vi "Autonomous Independent.vi"() -> ()   [LabVIEW 2014]
doc: "This VI is called when autonomous begins, and will automatically be terminated when autonomous ends. You can carry out timed or sensor driven robot movement independently without needing to return to the caller."
uses:
  Robot Global Data.vi
  <vilib>/Rock Robotics/WPI/RobotDrive/WPI_RobotDriveMecanumDrive_Cartesian.vi
  <vilib>/addons/control/pid/NI_PID_pid.lvlib
  <vilib>/addons/control/pid/pid.llb/PID (DBL).vi
  <vilib>/Rock Robotics/WPI/Relay/WPI_RelayValue.ctl
panel:
  out "Motor Outputs 2":dbl(graph)=0.07468179223935595
  in  "Target Center Gains":T1={"proportional gain (Kc)"=0.2, "integral time (Ti, min)"=0.0, "derivative time (Td, min)"=0.4} {"derivative time (Td, min)" format="%#.6g"; "integral time (Ti, min)" format="%#.6g"; "proportional gain (Kc)" format="%#.6g"}
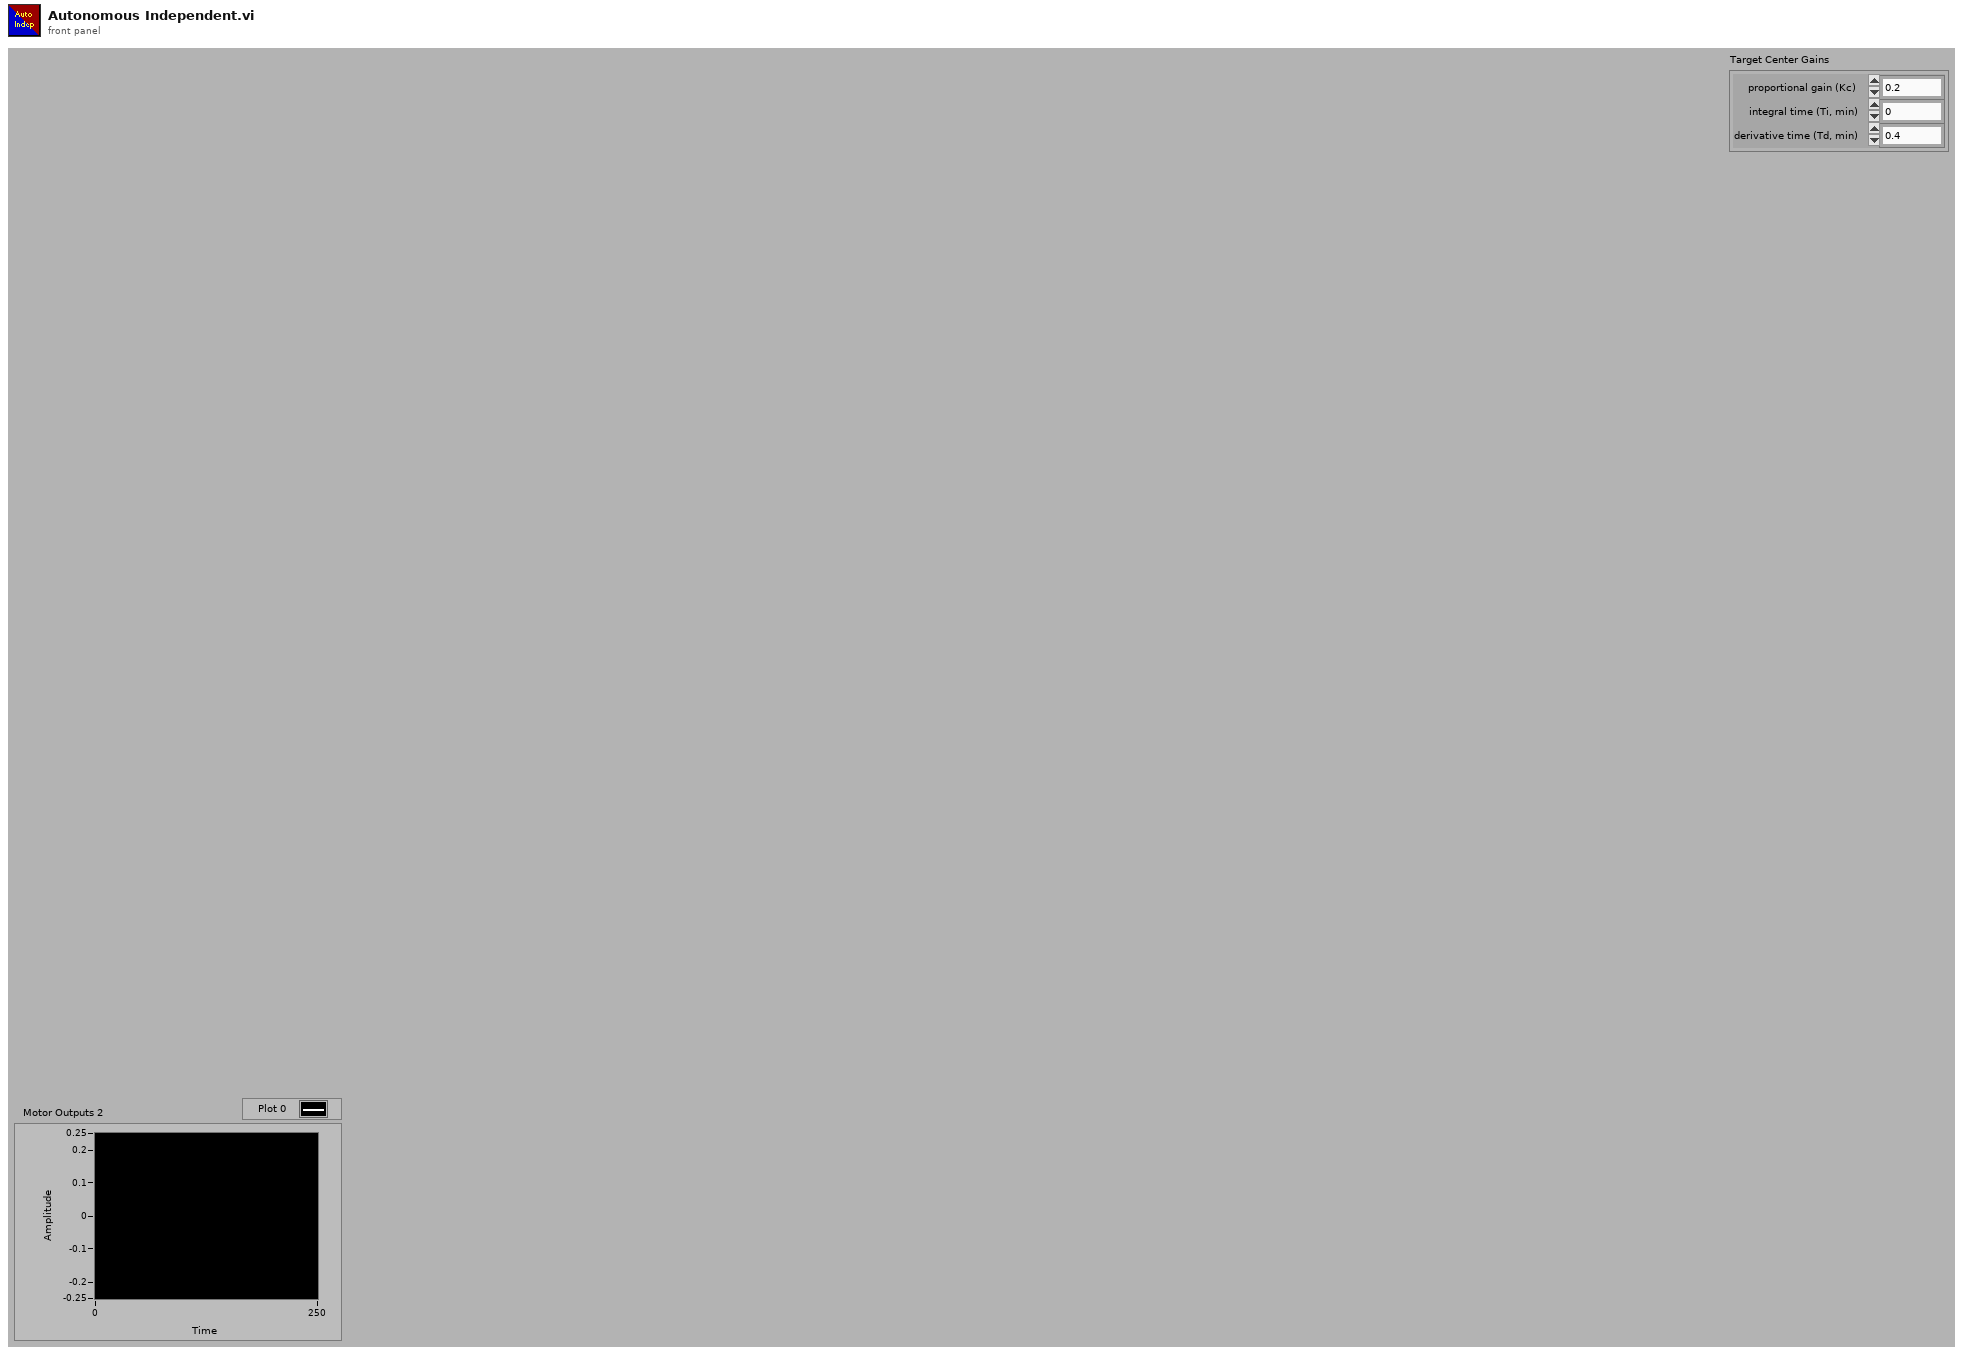
[diagram p1: front panel]
types:
  T1 = cluster{"proportional gain (Kc)":dbl, "integral time (Ti, min)":dbl, "derivative time (Td, min)":dbl}
  T2 = typedef "WPI_RelayValue.ctl" = enum16{"Off", "On", "Forward", "Reverse"}
  T3 = typedef "WPI_RelayDevRef.ctl" = cluster{"DevStatus":errorcluster, "Relay Channel":T4, "Digital Module":T5, "Relay Direction":T6}
  T4 = typedef "FPGA_DIORelayChannel.ctl" = enum8{"Relay 1", "Relay 2", "Relay 3", "Relay 4", "Relay 5", "Relay 6", "Relay 7", "Relay 8", "Invalid"}
  T5 = typedef "FPGA_TypedefDigitalModule.ctl" = enum16{"Digital Module 1", "Digital Module 2"}
  T6 = typedef "WPI_RelayDirection.ctl" = enum16{"Both directions", "Forward only", "Reverse only"}
  T7 = typedef "WPI_RobotDriveDevRef.ctl" = cluster{"DevStatus":errorcluster, "Motors[]":T8[], "Square Inputs":bool, "Max Output":dbl, "Isochronous":bool}
  T8 = typedef "WPI_MotorControlDeviceRef.ctl" = cluster{"DeviceStatus":errorcluster, "Type":enum16{"PWM", "CAN"}, "PWM":cluster{"Digital Module":T5, "PWM Channel":T9, "DeadBand":T10}, "CAN":cluster{"Device Number":u8, "Control Mode":T11, "Semaphore":T12, "Max Vout":dbl}, "Invert":bool, "TransformRef":T13, "InvTransformRef":T13}
  T9 = typedef "FPGA_DIOPWMChannel.ctl" = enum8{"PWM 1", "PWM 2", "PWM 3", "PWM 4", "PWM 5", "PWM 6", "PWM 7", "PWM 8", "PWM 9", "PWM 10", "Invalid"}
  T10 = typedef "WPI_PWMDeadband.ctl" = cluster{"Name":string, "maxPositivePwm":i32, "minPositivePwm":i32, "centerPwm":i32, "maxNegativePwm":i32, "minNegativePwm":i32, "angularRange":u16}
  T11 = typedef "WPI_CANJaguar_ControlMode.ctl" = enum8{"Percent VBus", "Current", "Speed", "Position", "Voltage"}
  T12 = typedef "Semaphore RefNum" = refnum<k1>
  T13 = typedef "WPI_PWMTransform_ConPane.ctl" = refnum<vi>
  T14 = typedef "WPI_JoystickDevRef.ctl" = cluster{"Device":T15}
  T15 = typedef "WPI_JoystickDeviceEnum.ctl" = enum16{"USB 1", "USB 2", "USB 3", "USB 4", "Kinect 1", "Kinect 2"}
  T16 = cluster{"axis 1 (x)":dbl, "axis 2 (y)":dbl, "axis 3 (throttle)":dbl, "axis 4":dbl, "axis 5":dbl, "axis 6":dbl}
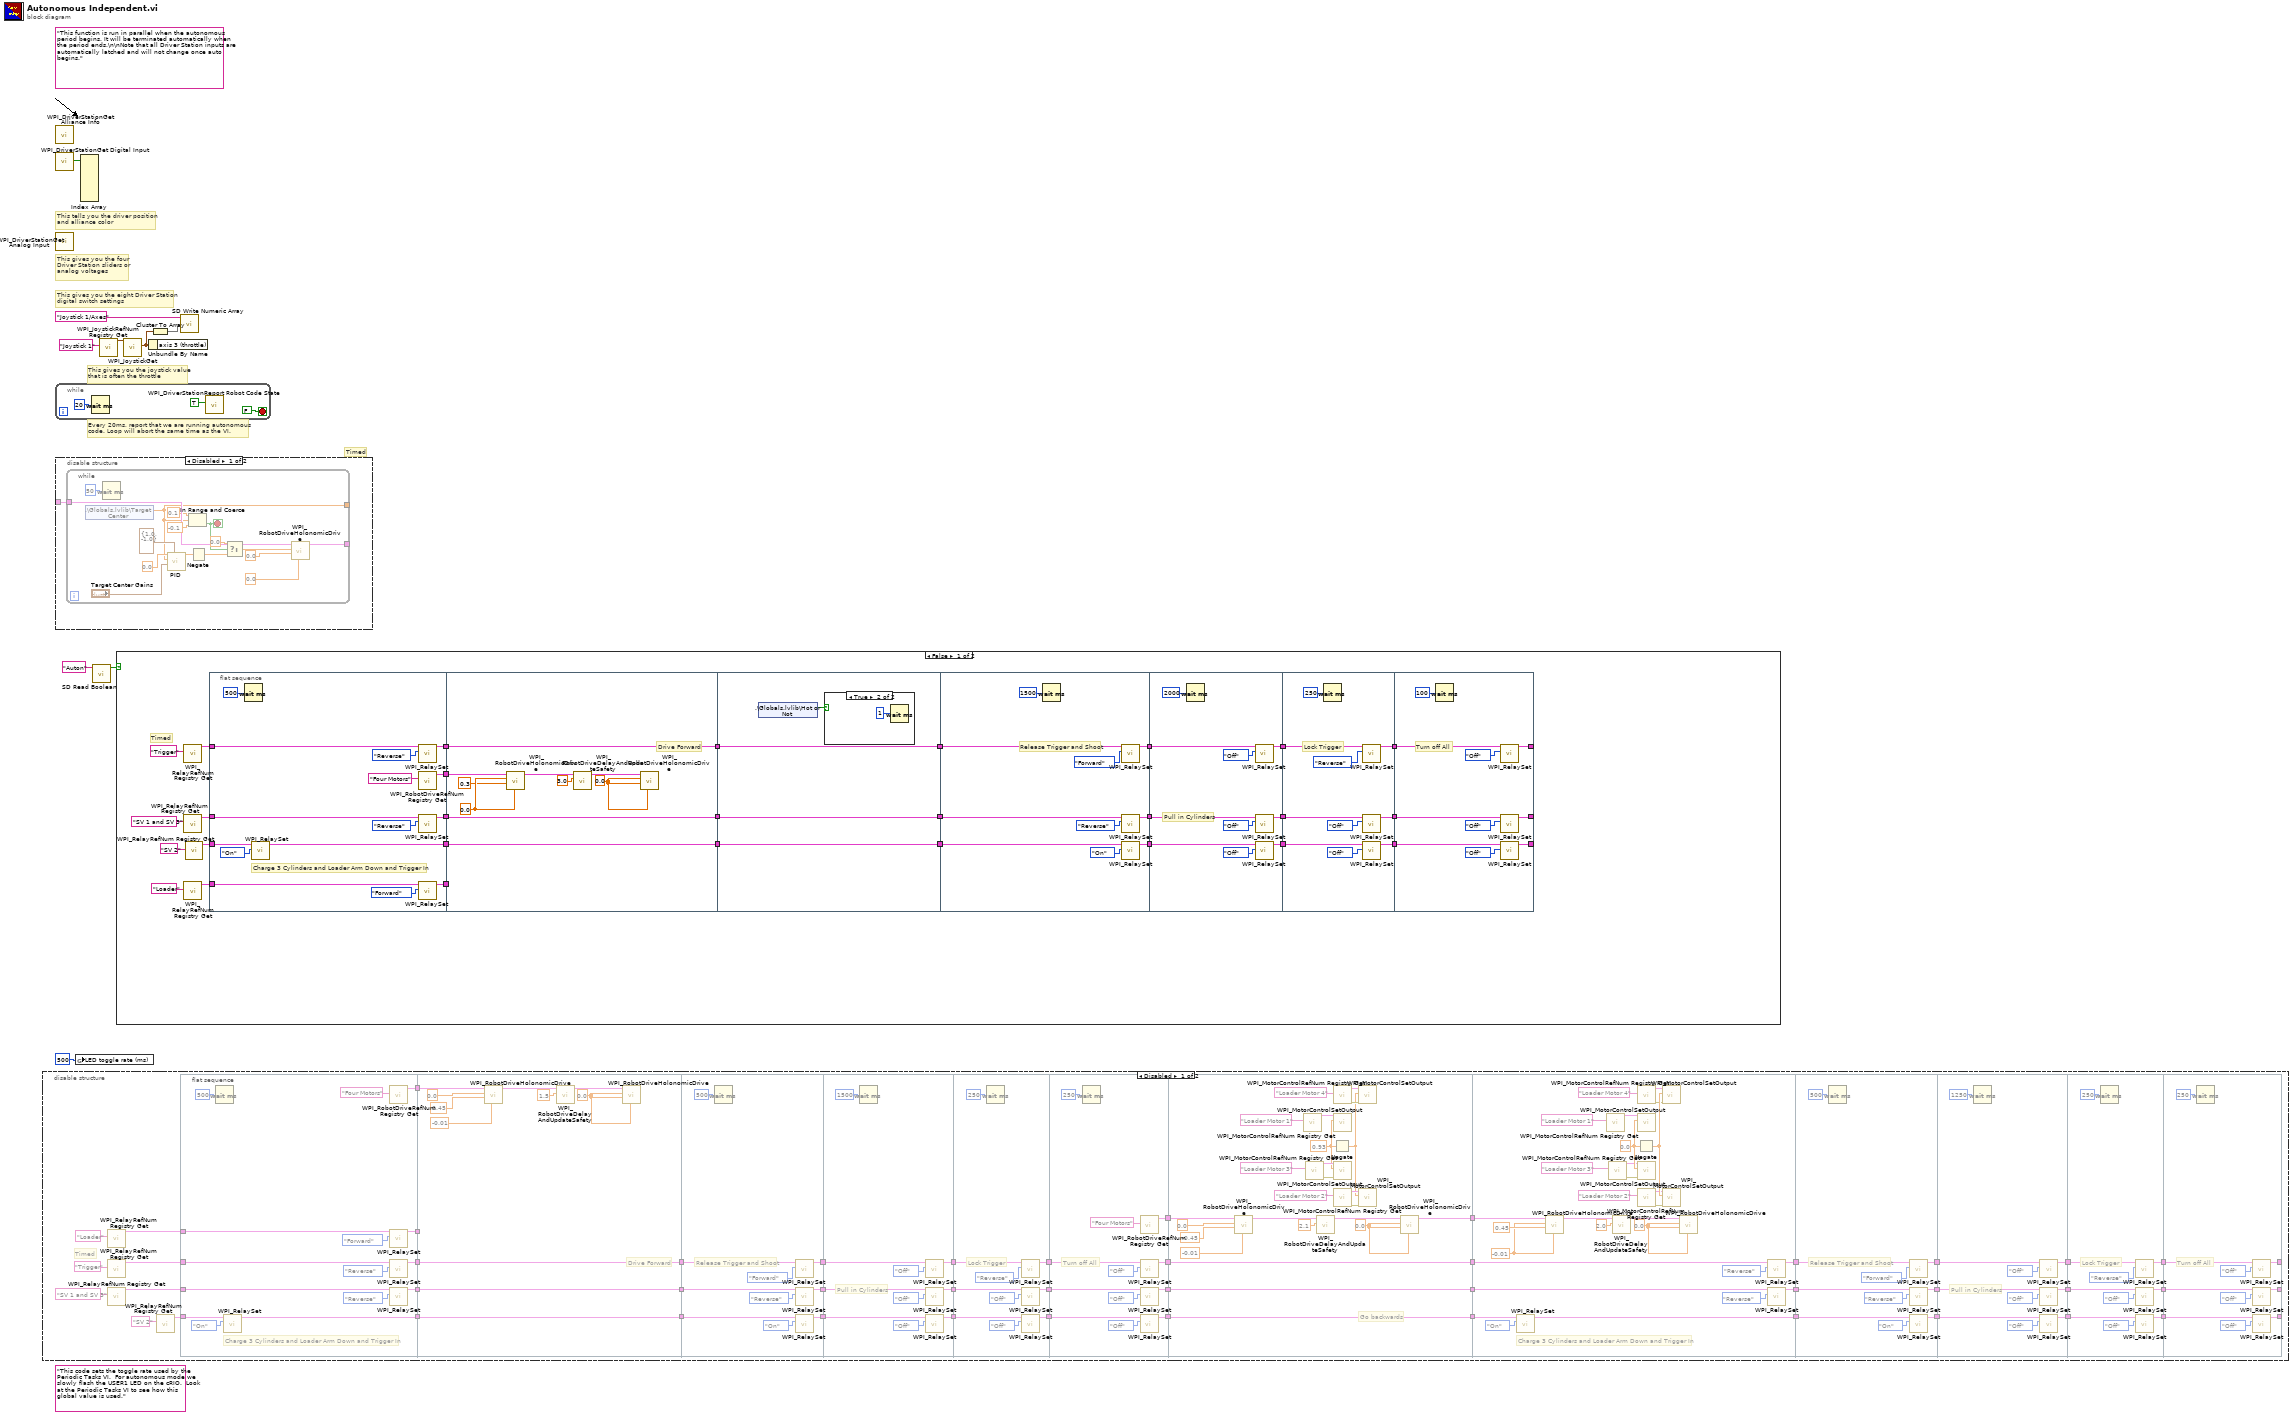
[diagram p0: block diagram]
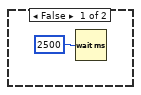
[diagram p2: hidden frame]
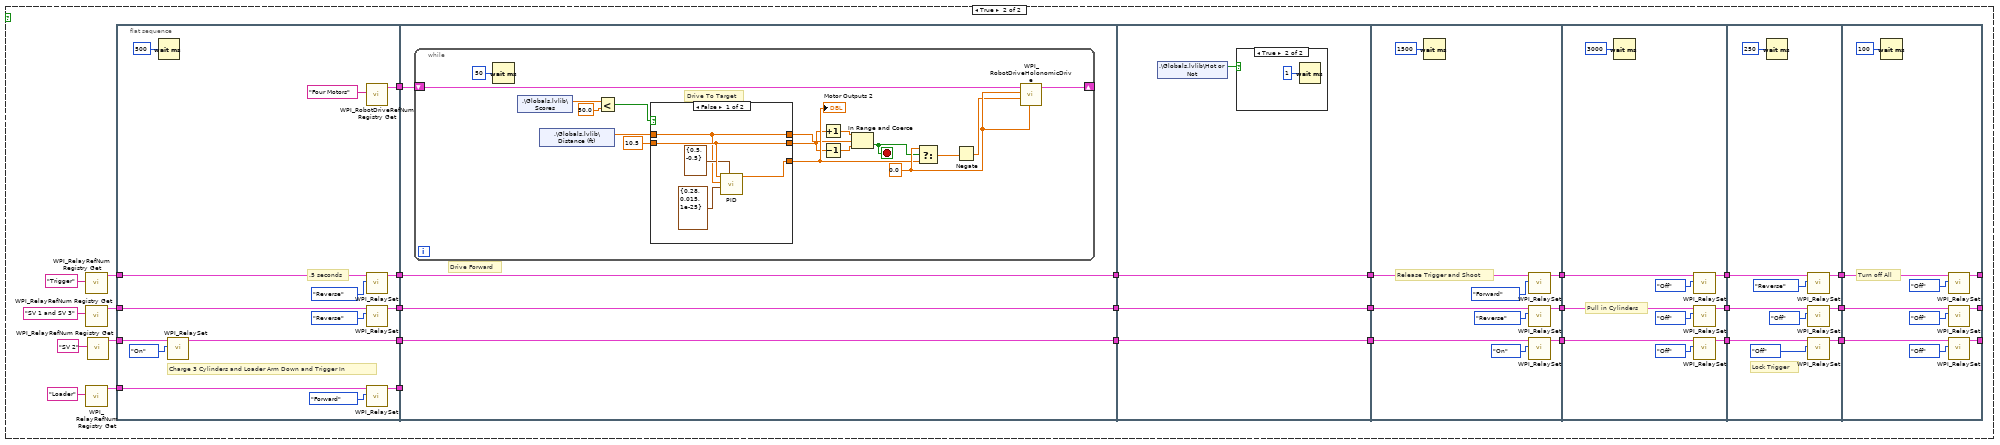
[diagram p3: hidden frame]
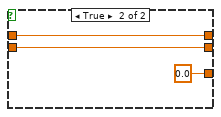
[diagram p4: hidden frame]
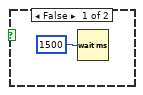
[diagram p5: hidden frame]
diagram:
  (unwired) "This code sets the toggle rate used by the Periodic Tasks VI.  For autonomous mode we slowly flash the USER1 LED on the cRIO.  Look at the Periodic Tasks VI to see how this global value is used."
  (unwired) "This function is run in parallel when the autonomous period begins. It will be terminated automatically when the period ends.\n\nNote that all Driver Station inputs are automatically latched and will not change once auto begins."
  # "Timed"
  # "Every 20ms, report that we are running autonomous\ncode. Loop will abort the same time as the VI."
  # "This gives you the joystick value\nthat is often the throttle"
  # "This tells you the driver position\nand alliance color"
  # "This gives you the eight Driver Station\ndigital switch settings"
  # "This gives you the four\nDriver Station sliders or\nanalog voltages"
  n1 = disable-structure shown="Disabled" {
    frame Disabled {
      # "Timed"
      n2 = call <vilib>:"WPI_RelayRefNum Registry Get.vi"("refnum name"="Loader") -> ("RelayDevRef"=w14:T3)  [unwired: 9 in, 1 out]
      n3 = call <vilib>:"WPI_RelayRefNum Registry Get.vi"("refnum name"="Trigger") -> ("RelayDevRef"=w16:T3)  [unwired: 9 in, 1 out]
      n4 = call <vilib>:"WPI_RelayRefNum Registry Get.vi"("refnum name"="SV 1 and SV 3") -> ("RelayDevRef"=w12:T3)  [unwired: 9 in, 1 out]
      n5 = call <vilib>:"WPI_RelayRefNum Registry Get.vi"("refnum name"="SV 2") -> ("RelayDevRef"=w10:T3)  [unwired: 9 in, 1 out]
      n6 = flat-sequence {
        tunnel: [w64] -> w54
        tunnel: [w63] -> w53
        tunnel: [w62] -> w52
        tunnel: [w61] -> w51
        tunnel: [w59] -> w50
        tunnel: w16 -> [w58]
        tunnel: w14 -> [w57]
        tunnel: w12 -> [w56]
        tunnel: w10 -> [w55]
        tunnel: w54 -> [_]
        tunnel: w53 -> [w80]
        tunnel: w52 -> [w79]
        tunnel: w51 -> [w78]
        tunnel: w50 -> [w73]
        tunnel: [w80] -> w47
        tunnel: [w79] -> w48
        tunnel: [w78] -> w49
        tunnel: [w83] -> w46
        tunnel: [w82] -> w45
        tunnel: [w81] -> w44
        tunnel: w49 -> [w84]
        tunnel: w48 -> [w85]
        tunnel: w47 -> [w86]
        tunnel: w46 -> [w96]
        tunnel: w45 -> [w95]
        tunnel: w44 -> [w94]
        tunnel: [w93] -> w43
        tunnel: [w92] -> w42
        tunnel: [w91] -> w41
        tunnel: w43 -> [w106]
        tunnel: w42 -> [w105]
        tunnel: w41 -> [w104]
        tunnel: [w103] -> w40
        tunnel: [w102] -> w39
        tunnel: [w101] -> w38
        tunnel: w40 -> [w118]
        tunnel: w39 -> [w117]
        tunnel: w38 -> [w116]
        tunnel: [w115] -> w37
        tunnel: [w114] -> w36
        tunnel: [w113] -> w35
        tunnel: [w111] -> w34
        tunnel: w37 -> [w147]
        tunnel: w36 -> [w146]
        tunnel: w35 -> [w145]
        tunnel: w34 -> [w138]
        tunnel: [w147] -> w30
        tunnel: [w146] -> w31
        tunnel: [w145] -> w32
        tunnel: [w124] -> w33
        tunnel: [w176] -> w29
        tunnel: [w175] -> w28
        tunnel: [w174] -> w27
        tunnel: w33 -> [w150]
        tunnel: w32 -> [w155]
        tunnel: w31 -> [w156]
        tunnel: w30 -> [w157]
        tunnel: w29 -> [w180]
        tunnel: w28 -> [w182]
        tunnel: w27 -> [w178]
        tunnel: [w181] -> w26
        tunnel: [w179] -> w25
        tunnel: [w177] -> w24
        tunnel: w26 -> [w192]
        tunnel: w25 -> [w191]
        tunnel: w24 -> [w190]
        tunnel: [w189] -> w23
        tunnel: [w188] -> w22
        tunnel: [w187] -> w21
        tunnel: w23 -> [w202]
        tunnel: w22 -> [w201]
        tunnel: w21 -> [w200]
        tunnel: [w199] -> w20
        tunnel: [w198] -> w19
        tunnel: [w197] -> w18
        tunnel: w20 -> [w212]
        tunnel: w19 -> [w211]
        tunnel: w18 -> [w210]
        tunnel: [w209] -> _
        tunnel: [w208] -> _
        tunnel: [w207] -> _
        frame #0 {
          # "Charge 3 Cylinders and Loader Arm Down and Trigger In"
          n7 = Wait (ms)(milliseconds to wait=u32 500) -> ()  [unwired: 1 out]
          n8 = call <vilib>:"WPI_RelaySet.vi"("RelayValue"=WPI_RelayValue."On", "RelayDevRef"=w55) -> ("RelayDevRef"=w63:T3)  [unwired: 8 in, 1 out]
          n9 = call <vilib>:"WPI_RobotDriveRefNum Registry Get.vi"("refnum name"="Four Motors") -> ("RobotDriveDevRef"=w59:T7)  [unwired: 1 in, 9 out]
          n10 = call <vilib>:"WPI_RelaySet.vi"("RelayValue"=WPI_RelayValue."Forward", "RelayDevRef"=w57) -> ("RelayDevRef"=w64:T3)  [unwired: 8 in, 1 out]
          n11 = call <vilib>:"WPI_RelaySet.vi"("RelayValue"=WPI_RelayValue."Reverse", "RelayDevRef"=w58) -> ("RelayDevRef"=w62:T3)  [unwired: 8 in, 1 out]
          n12 = call <vilib>:"WPI_RelaySet.vi"("RelayValue"=WPI_RelayValue."Reverse", "RelayDevRef"=w56) -> ("RelayDevRef"=w61:T3)  [unwired: 8 in, 1 out]
        }
        frame #1 {
          w74 = 0.0 ("Y")
          # "Drive Forward"
          n13 = call-poly <vilib>:"WPI_RobotDriveHolonomicDrive.vi"("Rotation"=-0.01, "Y"=0.45, "X"=0.0 ("Y"), "RobotDriveDevRef"=w73) -> ("RobotDriveDevRef"=w77:T7)  [unwired: 5 in, 2 out]
          n14 = call <vilib>:"WPI_RobotDriveDelayAndUpdateSafety.vi"("Delay (s)"=1.5, "RobotDriveDevRef"=w77) -> ("RobotDriveDevRef 2"=w75:T7)  [unwired: 8 in, 1 out]
          n15 = call-poly <vilib>:"WPI_RobotDriveHolonomicDrive.vi"("Rotation"=w74, "Y"=w74, "X"=w74, "RobotDriveDevRef"=w75) -> ()  [unwired: 5 in, 3 out]
        }
        frame #2 {
          # "Release Trigger and Shoot"
          n16 = Wait (ms)(milliseconds to wait=u32 500) -> ()  [unwired: 1 out]
          n17 = call <vilib>:"WPI_RelaySet.vi"("RelayValue"=WPI_RelayValue."Forward", "RelayDevRef"=w85) -> ("RelayDevRef"=w82:T3)  [unwired: 8 in, 1 out]
          n18 = call <vilib>:"WPI_RelaySet.vi"("RelayValue"=WPI_RelayValue."Reverse", "RelayDevRef"=w84) -> ("RelayDevRef"=w81:T3)  [unwired: 8 in, 1 out]
          n19 = call <vilib>:"WPI_RelaySet.vi"("RelayValue"=WPI_RelayValue."On", "RelayDevRef"=w86) -> ("RelayDevRef"=w83:T3)  [unwired: 8 in, 1 out]
        }
        frame #3 {
          # "Pull in Cylinders"
          n20 = Wait (ms)(milliseconds to wait=u32 1500) -> ()  [unwired: 1 out]
          n21 = call <vilib>:"WPI_RelaySet.vi"("RelayValue"=WPI_RelayValue."Off", "RelayDevRef"=w95) -> ("RelayDevRef"=w92:T3)  [unwired: 8 in, 1 out]
          n22 = call <vilib>:"WPI_RelaySet.vi"("RelayValue"=WPI_RelayValue."Off", "RelayDevRef"=w94) -> ("RelayDevRef"=w91:T3)  [unwired: 8 in, 1 out]
          n23 = call <vilib>:"WPI_RelaySet.vi"("RelayValue"=WPI_RelayValue."Off", "RelayDevRef"=w96) -> ("RelayDevRef"=w93:T3)  [unwired: 8 in, 1 out]
        }
        frame #4 {
          # "Lock Trigger"
          n24 = Wait (ms)(milliseconds to wait=u32 250) -> ()  [unwired: 1 out]
          n25 = call <vilib>:"WPI_RelaySet.vi"("RelayValue"=WPI_RelayValue."Reverse", "RelayDevRef"=w105) -> ("RelayDevRef"=w102:T3)  [unwired: 8 in, 1 out]
          n26 = call <vilib>:"WPI_RelaySet.vi"("RelayValue"=WPI_RelayValue."Off", "RelayDevRef"=w104) -> ("RelayDevRef"=w101:T3)  [unwired: 8 in, 1 out]
          n27 = call <vilib>:"WPI_RelaySet.vi"("RelayValue"=WPI_RelayValue."Off", "RelayDevRef"=w106) -> ("RelayDevRef"=w103:T3)  [unwired: 8 in, 1 out]
        }
        frame #5 {
          # "Turn off All"
          n28 = Wait (ms)(milliseconds to wait=u32 250) -> ()  [unwired: 1 out]
          n29 = call <vilib>:"WPI_RobotDriveRefNum Registry Get.vi"("refnum name"="Four Motors") -> ("RobotDriveDevRef"=w111:T7)  [unwired: 1 in, 9 out]
          n30 = call <vilib>:"WPI_RelaySet.vi"("RelayValue"=WPI_RelayValue."Off", "RelayDevRef"=w117) -> ("RelayDevRef"=w114:T3)  [unwired: 8 in, 1 out]
          n31 = call <vilib>:"WPI_RelaySet.vi"("RelayValue"=WPI_RelayValue."Off", "RelayDevRef"=w116) -> ("RelayDevRef"=w115:T3)  [unwired: 8 in, 1 out]
          n32 = call <vilib>:"WPI_RelaySet.vi"("RelayValue"=WPI_RelayValue."Off", "RelayDevRef"=w118) -> ("RelayDevRef"=w113:T3)  [unwired: 8 in, 1 out]
        }
        frame #6 {
          w125 = 0.93 ("t")
          w141 = 0.0 ("Y")
          # "Go backwards"
          n33 = call-poly <vilib>:"WPI_RobotDriveHolonomicDrive.vi"("Rotation"=-0.01, "Y"=-0.45, "X"=0.0 ("Y"), "RobotDriveDevRef"=w138) -> ("RobotDriveDevRef"=w144:T7)  [unwired: 5 in, 2 out]
          n34 = call <vilib>:"WPI_MotorControlRefNum Registry Get.vi"("refnum name"="Loader Motor 1") -> ("MotorControlDevRef"=w134:T8)  [unwired: 9 in, 1 out]
          n35 = call <vilib>:"WPI_MotorControlRefNum Registry Get.vi"("refnum name"="Loader Motor 3") -> ("error out"=w130:errorcluster, "MotorControlDevRef"=w131:T8)  [unwired: 9 in]
          n36 = call <vilib>:"WPI_RobotDriveDelayAndUpdateSafety.vi"("Delay (s)"=2.1, "RobotDriveDevRef"=w144) -> ("RobotDriveDevRef 2"=w142:T7)  [unwired: 8 in, 1 out]
          n37 = call <vilib>:"WPI_MotorControlRefNum Registry Get.vi"("refnum name"="Loader Motor 4") -> ("error out"=w127:errorcluster, "MotorControlDevRef"=w128:T8)  [unwired: 9 in]
          n38 = call <vilib>:"WPI_MotorControlSetOutput.vi"("Output"=w125, "MotorControlDevRef"=w134) -> ()  [unwired: 7 in, 3 out]
          n39 = Negate(x=w125) -> (-x=w126:dbl)
          n40 = call <vilib>:"WPI_MotorControlSetOutput.vi"("error in (no error)"=w130, "Output"=w125, "MotorControlDevRef"=w131) -> ()  [unwired: 6 in, 3 out]
          n41 = call <vilib>:"WPI_MotorControlRefNum Registry Get.vi"("refnum name"="Loader Motor 2") -> ("error out"=w133:errorcluster, "MotorControlDevRef"=w135:T8)  [unwired: 9 in]
          n42 = call <vilib>:"WPI_MotorControlSetOutput.vi"("error in (no error)"=w127, "Output"=w126, "MotorControlDevRef"=w128) -> ()  [unwired: 6 in, 3 out]
          n43 = call <vilib>:"WPI_MotorControlSetOutput.vi"("error in (no error)"=w133, "Output"=w126, "MotorControlDevRef"=w135) -> ()  [unwired: 6 in, 3 out]
          n44 = call-poly <vilib>:"WPI_RobotDriveHolonomicDrive.vi"("Rotation"=w141, "Y"=w141, "X"=w141, "RobotDriveDevRef"=w142) -> ("RobotDriveDevRef"=w124:T7)  [unwired: 5 in, 2 out]
        }
        frame #7 {
          w148 = -0.01 ("Y")
          w149 = 0.0 ("Y")
          w173 = 0.0 ("t")
          # "Charge 3 Cylinders and Loader Arm Down and Trigger In"
          n45 = call <vilib>:"WPI_RelaySet.vi"("RelayValue"=WPI_RelayValue."On", "RelayDevRef"=w155) -> ("RelayDevRef"=w174:T3)  [unwired: 8 in, 1 out]
          n46 = call-poly <vilib>:"WPI_RobotDriveHolonomicDrive.vi"("Rotation"=w148, "Y"=0.45, "X"=w148, "RobotDriveDevRef"=w150) -> ("RobotDriveDevRef"=w151:T7)  [unwired: 5 in, 2 out]
          n47 = call <vilib>:"WPI_MotorControlRefNum Registry Get.vi"("refnum name"="Loader Motor 1") -> ("MotorControlDevRef"=w165:T8)  [unwired: 9 in, 1 out]
          n48 = call <vilib>:"WPI_MotorControlRefNum Registry Get.vi"("refnum name"="Loader Motor 3") -> ("error out"=w169:errorcluster, "MotorControlDevRef"=w168:T8)  [unwired: 9 in]
          n49 = call <vilib>:"WPI_RobotDriveDelayAndUpdateSafety.vi"("Delay (s)"=2.0, "RobotDriveDevRef"=w151) -> ("RobotDriveDevRef 2"=w153:T7)  [unwired: 8 in, 1 out]
          n50 = call <vilib>:"WPI_MotorControlRefNum Registry Get.vi"("refnum name"="Loader Motor 4") -> ("error out"=w171:errorcluster, "MotorControlDevRef"=w161:T8)  [unwired: 9 in]
          n51 = call <vilib>:"WPI_MotorControlSetOutput.vi"("Output"=w173, "MotorControlDevRef"=w165) -> ()  [unwired: 7 in, 3 out]
          n52 = Negate(x=w173) -> (-x=w172:dbl)
          n53 = call <vilib>:"WPI_MotorControlSetOutput.vi"("error in (no error)"=w169, "Output"=w173, "MotorControlDevRef"=w168) -> ()  [unwired: 6 in, 3 out]
          n54 = call <vilib>:"WPI_MotorControlRefNum Registry Get.vi"("refnum name"="Loader Motor 2") -> ("error out"=w166:errorcluster, "MotorControlDevRef"=w164:T8)  [unwired: 9 in]
          n55 = call <vilib>:"WPI_MotorControlSetOutput.vi"("error in (no error)"=w171, "Output"=w172, "MotorControlDevRef"=w161) -> ()  [unwired: 6 in, 3 out]
          n56 = call <vilib>:"WPI_MotorControlSetOutput.vi"("error in (no error)"=w166, "Output"=w172, "MotorControlDevRef"=w164) -> ()  [unwired: 6 in, 3 out]
          n57 = call-poly <vilib>:"WPI_RobotDriveHolonomicDrive.vi"("Rotation"=w149, "Y"=w149, "X"=w149, "RobotDriveDevRef"=w153) -> ()  [unwired: 5 in, 3 out]
          n58 = call <vilib>:"WPI_RelaySet.vi"("RelayValue"=WPI_RelayValue."Reverse", "RelayDevRef"=w156) -> ("RelayDevRef"=w175:T3)  [unwired: 8 in, 1 out]
          n59 = call <vilib>:"WPI_RelaySet.vi"("RelayValue"=WPI_RelayValue."Reverse", "RelayDevRef"=w157) -> ("RelayDevRef"=w176:T3)  [unwired: 8 in, 1 out]
        }
        frame #8 {
          # "Release Trigger and Shoot"
          n60 = Wait (ms)(milliseconds to wait=u32 500) -> ()  [unwired: 1 out]
          n61 = call <vilib>:"WPI_RelaySet.vi"("RelayValue"=WPI_RelayValue."Forward", "RelayDevRef"=w182) -> ("RelayDevRef"=w181:T3)  [unwired: 8 in, 1 out]
          n62 = call <vilib>:"WPI_RelaySet.vi"("RelayValue"=WPI_RelayValue."Reverse", "RelayDevRef"=w180) -> ("RelayDevRef"=w179:T3)  [unwired: 8 in, 1 out]
          n63 = call <vilib>:"WPI_RelaySet.vi"("RelayValue"=WPI_RelayValue."On", "RelayDevRef"=w178) -> ("RelayDevRef"=w177:T3)  [unwired: 8 in, 1 out]
        }
        frame #9 {
          # "Pull in Cylinders"
          n64 = Wait (ms)(milliseconds to wait=u32 1250) -> ()  [unwired: 1 out]
          n65 = call <vilib>:"WPI_RelaySet.vi"("RelayValue"=WPI_RelayValue."Off", "RelayDevRef"=w192) -> ("RelayDevRef"=w189:T3)  [unwired: 8 in, 1 out]
          n66 = call <vilib>:"WPI_RelaySet.vi"("RelayValue"=WPI_RelayValue."Off", "RelayDevRef"=w191) -> ("RelayDevRef"=w188:T3)  [unwired: 8 in, 1 out]
          n67 = call <vilib>:"WPI_RelaySet.vi"("RelayValue"=WPI_RelayValue."Off", "RelayDevRef"=w190) -> ("RelayDevRef"=w187:T3)  [unwired: 8 in, 1 out]
        }
        frame #10 {
          # "Lock Trigger"
          n68 = Wait (ms)(milliseconds to wait=u32 250) -> ()  [unwired: 1 out]
          n69 = call <vilib>:"WPI_RelaySet.vi"("RelayValue"=WPI_RelayValue."Reverse", "RelayDevRef"=w202) -> ("RelayDevRef"=w199:T3)  [unwired: 8 in, 1 out]
          n70 = call <vilib>:"WPI_RelaySet.vi"("RelayValue"=WPI_RelayValue."Off", "RelayDevRef"=w201) -> ("RelayDevRef"=w198:T3)  [unwired: 8 in, 1 out]
          n71 = call <vilib>:"WPI_RelaySet.vi"("RelayValue"=WPI_RelayValue."Off", "RelayDevRef"=w200) -> ("RelayDevRef"=w197:T3)  [unwired: 8 in, 1 out]
        }
        frame #11 {
          # "Turn off All"
          n72 = Wait (ms)(milliseconds to wait=u32 250) -> ()  [unwired: 1 out]
          n73 = call <vilib>:"WPI_RelaySet.vi"("RelayValue"=WPI_RelayValue."Off", "RelayDevRef"=w212) -> ("RelayDevRef"=w208:T3)  [unwired: 8 in, 1 out]
          n74 = call <vilib>:"WPI_RelaySet.vi"("RelayValue"=WPI_RelayValue."Off", "RelayDevRef"=w211) -> ("RelayDevRef"=w209:T3)  [unwired: 8 in, 1 out]
          n75 = call <vilib>:"WPI_RelaySet.vi"("RelayValue"=WPI_RelayValue."Off", "RelayDevRef"=w210) -> ("RelayDevRef"=w207:T3)  [unwired: 8 in, 1 out]
        }
      }
    }
    frame Enabled {
    }
  }
  n76 = call <vilib>:"WPI_DriverStationGet Alliance Info.vi"() -> ()  [unwired: 12 out]
  n77 = call <vilib>:"WPI_DriverStationGet Digital Input.vi"() -> ("Driver Station Digital Input (1-8)"=w9:bool[])  [unwired: 11 out]
  n78 = call <vilib>:"WPI_DriverStationGet Analog Input.vi"() -> ()  [unwired: 12 out]
  n79 = while {
    stop <- FALSE stop-if-true
    n80 = Wait (ms)(milliseconds to wait=u32 20) -> ()  [unwired: 1 out]
    n81 = call <vilib>:"WPI_DriverStationReport Robot Code State.vi"("Autonomous"=TRUE) -> ()  [unwired: 10 in, 1 out]
  }
  n82 = disable-structure shown="Disabled" {
    disable-tunnel: _ -> [w220 _]
    frame Disabled {
      n83 = while {
        tunnel: w220 -> [w236]
        tunnel: [w224] -> _
        tunnel: [w223] -> _
        stop <- w222 stop-if-true
        n84 = shared-variable ".\\Globals.lvlib\\Target Center"() -> (w224:dbl)  [unwired: 1 in, 1 out]
        n85 = Wait (ms)(milliseconds to wait=u32 50) -> ()  [unwired: 1 out]
        n86 = call-poly <vilib>:"PID.vi"("output range"=cluster{"output high":dbl, "output low":dbl} {"output high"=1.0, "output low"=-1.0}, "PID gains"="Target Center Gains", "process variable"=w224, "setpoint"=0.0) -> ("output"=w231:dbl)  [unwired: 6 in, 1 out]
        n87 = In Range and Coerce(upper limit=0.1, x=w224, lower limit=-0.1) -> (In Range?=w222:bool)  [unwired: 1 out]
        n88 = Negate(x=w231) -> (-x=w227:dbl)
        n89 = Select(t=0.0, s=w222, f=w227) -> (s? t:f=w226:dbl)
        n90 = call-poly <vilib>:"WPI_RobotDriveHolonomicDrive.vi"("Rotation"=0.0 ("Y"), "Y"=0.0, "X"=w226, "RobotDriveDevRef"=w236) -> ("RobotDriveDevRef"=w223:T7)  [unwired: 5 in, 2 out]
      }
    }
    frame Enabled {
    }
  }
  n91 = global write "Robot Global Data.vi" "LED toggle rate (ms)"(u32 500 ("LED ms toggle rate")) -> ()
  n92 = Index Array(array=w9) -> ()  [unwired: 8 in, 8 out]
  n93 = call <vilib>:"SD Read Boolean.vi"("Name"="Auton") -> ("Boolean"=w1:bool)  [unwired: 8 in, 2 out]
  n94 = call <vilib>:"WPI_JoystickRefNum Registry Get.vi"("refnum name"="Joystick 1") -> ("JoystickDevRef"=w7:T14)  [unwired: 1 in, 9 out]
  n95 = case shown="False" w1 {
    frame False {
      # "Timed"
      n96 = call <vilib>:"WPI_RelayRefNum Registry Get.vi"("refnum name"="Trigger") -> ("RelayDevRef"=w243:T3)  [unwired: 9 in, 1 out]
      n97 = call <vilib>:"WPI_RelayRefNum Registry Get.vi"("refnum name"="SV 1 and SV 3") -> ("RelayDevRef"=w239:T3)  [unwired: 9 in, 1 out]
      n98 = call <vilib>:"WPI_RelayRefNum Registry Get.vi"("refnum name"="Loader") -> ("RelayDevRef"=w241:T3)  [unwired: 9 in, 1 out]
      n99 = call <vilib>:"WPI_RelayRefNum Registry Get.vi"("refnum name"="SV 2") -> ("RelayDevRef"=w237:T3)  [unwired: 9 in, 1 out]
      n100 = flat-sequence {
        tunnel: [w274] -> w264
        tunnel: [w273] -> w263
        tunnel: [w272] -> w262
        tunnel: [w271] -> w261
        tunnel: [w269] -> w260
        tunnel: w243 -> [w268]
        tunnel: w241 -> [w267]
        tunnel: w239 -> [w266]
        tunnel: w237 -> [w265]
        tunnel: w264 -> [_]
        tunnel: w263 -> [w289]
        tunnel: w262 -> [w288]
        tunnel: w261 -> [w287]
        tunnel: w260 -> [w282]
        tunnel: [w289] -> w259
        tunnel: [w288] -> w258
        tunnel: [w287] -> w257
        tunnel: w259 -> [w293]
        tunnel: w258 -> [w292]
        tunnel: w257 -> [w291]
        tunnel: [w293] -> w256
        tunnel: [w292] -> w255
        tunnel: [w291] -> w254
        tunnel: w256 -> [w301]
        tunnel: w255 -> [w300]
        tunnel: w254 -> [w299]
        tunnel: [w298] -> w253
        tunnel: [w297] -> w252
        tunnel: [w296] -> w251
        tunnel: w253 -> [w311]
        tunnel: w252 -> [w310]
        tunnel: w251 -> [w309]
        tunnel: [w308] -> w250
        tunnel: [w307] -> w249
        tunnel: [w306] -> w248
        tunnel: w250 -> [w321]
        tunnel: w249 -> [w320]
        tunnel: w248 -> [w319]
        tunnel: [w318] -> w247
        tunnel: [w317] -> w246
        tunnel: [w316] -> w245
        tunnel: w247 -> [w331]
        tunnel: w246 -> [w330]
        tunnel: w245 -> [w329]
        tunnel: [w328] -> _
        tunnel: [w327] -> _
        tunnel: [w326] -> _
        frame #0 {
          # "Charge 3 Cylinders and Loader Arm Down and Trigger In"
          n101 = Wait (ms)(milliseconds to wait=u32 500) -> ()  [unwired: 1 out]
          n102 = call <vilib>:"WPI_RelaySet.vi"("RelayValue"=WPI_RelayValue."On", "RelayDevRef"=w265) -> ("RelayDevRef"=w273:T3)  [unwired: 8 in, 1 out]
          n103 = call <vilib>:"WPI_RelaySet.vi"("RelayValue"=WPI_RelayValue."Reverse", "RelayDevRef"=w268) -> ("RelayDevRef"=w272:T3)  [unwired: 8 in, 1 out]
          n104 = call <vilib>:"WPI_RobotDriveRefNum Registry Get.vi"("refnum name"="Four Motors") -> ("RobotDriveDevRef"=w269:T7)  [unwired: 1 in, 9 out]
          n105 = call <vilib>:"WPI_RelaySet.vi"("RelayValue"=WPI_RelayValue."Reverse", "RelayDevRef"=w266) -> ("RelayDevRef"=w271:T3)  [unwired: 8 in, 1 out]
          n106 = call <vilib>:"WPI_RelaySet.vi"("RelayValue"=WPI_RelayValue."Forward", "RelayDevRef"=w267) -> ("RelayDevRef"=w274:T3)  [unwired: 8 in, 1 out]
        }
        frame #1 {
          w281 = 0.0 ("Y")
          w283 = 0.0 ("Y")
          # "Drive Forward"
          n107 = call-poly <vilib>:"WPI_RobotDriveHolonomicDrive.vi"("Rotation"=w281, "Y"=0.3, "X"=w281, "RobotDriveDevRef"=w282) -> ("RobotDriveDevRef"=w286:T7)  [unwired: 5 in, 2 out]
          n108 = call <vilib>:"WPI_RobotDriveDelayAndUpdateSafety.vi"("Delay (s)"=3.0, "RobotDriveDevRef"=w286) -> ("RobotDriveDevRef 2"=w284:T7)  [unwired: 8 in, 1 out]
          n109 = call-poly <vilib>:"WPI_RobotDriveHolonomicDrive.vi"("Rotation"=w283, "Y"=w283, "X"=w283, "RobotDriveDevRef"=w284) -> ()  [unwired: 5 in, 3 out]
        }
        frame #2 {
          n110 = shared-variable ".\\Globals.lvlib\\Hot or Not"() -> (w290:bool)  [unwired: 1 in, 1 out]
          n111 = case shown="True" w290 {
            frame False {
              n112 = Wait (ms)(milliseconds to wait=u32 2500) -> ()  [unwired: 1 out]
            }
            frame True {
              n113 = Wait (ms)(milliseconds to wait=u32 1) -> ()  [unwired: 1 out]
            }
          }
        }
        frame #3 {
          # "Release Trigger and Shoot"
          n114 = Wait (ms)(milliseconds to wait=u32 1500) -> ()  [unwired: 1 out]
          n115 = call <vilib>:"WPI_RelaySet.vi"("RelayValue"=WPI_RelayValue."Forward", "RelayDevRef"=w300) -> ("RelayDevRef"=w297:T3)  [unwired: 8 in, 1 out]
          n116 = call <vilib>:"WPI_RelaySet.vi"("RelayValue"=WPI_RelayValue."Reverse", "RelayDevRef"=w299) -> ("RelayDevRef"=w296:T3)  [unwired: 8 in, 1 out]
          n117 = call <vilib>:"WPI_RelaySet.vi"("RelayValue"=WPI_RelayValue."On", "RelayDevRef"=w301) -> ("RelayDevRef"=w298:T3)  [unwired: 8 in, 1 out]
        }
        frame #4 {
          # "Pull in Cylinders"
          n118 = Wait (ms)(milliseconds to wait=u32 2000) -> ()  [unwired: 1 out]
          n119 = call <vilib>:"WPI_RelaySet.vi"("RelayValue"=WPI_RelayValue."Off", "RelayDevRef"=w310) -> ("RelayDevRef"=w307:T3)  [unwired: 8 in, 1 out]
          n120 = call <vilib>:"WPI_RelaySet.vi"("RelayValue"=WPI_RelayValue."Off", "RelayDevRef"=w309) -> ("RelayDevRef"=w306:T3)  [unwired: 8 in, 1 out]
          n121 = call <vilib>:"WPI_RelaySet.vi"("RelayValue"=WPI_RelayValue."Off", "RelayDevRef"=w311) -> ("RelayDevRef"=w308:T3)  [unwired: 8 in, 1 out]
        }
        frame #5 {
          # "Lock Trigger"
          n122 = Wait (ms)(milliseconds to wait=u32 250) -> ()  [unwired: 1 out]
          n123 = call <vilib>:"WPI_RelaySet.vi"("RelayValue"=WPI_RelayValue."Reverse", "RelayDevRef"=w320) -> ("RelayDevRef"=w317:T3)  [unwired: 8 in, 1 out]
          n124 = call <vilib>:"WPI_RelaySet.vi"("RelayValue"=WPI_RelayValue."Off", "RelayDevRef"=w319) -> ("RelayDevRef"=w316:T3)  [unwired: 8 in, 1 out]
          n125 = call <vilib>:"WPI_RelaySet.vi"("RelayValue"=WPI_RelayValue."Off", "RelayDevRef"=w321) -> ("RelayDevRef"=w318:T3)  [unwired: 8 in, 1 out]
        }
        frame #6 {
          # "Turn off All"
          n126 = Wait (ms)(milliseconds to wait=u32 100) -> ()  [unwired: 1 out]
          n127 = call <vilib>:"WPI_RelaySet.vi"("RelayValue"=WPI_RelayValue."Off", "RelayDevRef"=w330) -> ("RelayDevRef"=w327:T3)  [unwired: 8 in, 1 out]
          n128 = call <vilib>:"WPI_RelaySet.vi"("RelayValue"=WPI_RelayValue."Off", "RelayDevRef"=w329) -> ("RelayDevRef"=w328:T3)  [unwired: 8 in, 1 out]
          n129 = call <vilib>:"WPI_RelaySet.vi"("RelayValue"=WPI_RelayValue."Off", "RelayDevRef"=w331) -> ("RelayDevRef"=w326:T3)  [unwired: 8 in, 1 out]
        }
      }
    }
    frame True {
      n130 = call <vilib>:"WPI_RelayRefNum Registry Get.vi"("refnum name"="Trigger") -> ("RelayDevRef"=w342:T3)  [unwired: 9 in, 1 out]
      n131 = call <vilib>:"WPI_RelayRefNum Registry Get.vi"("refnum name"="SV 1 and SV 3") -> ("RelayDevRef"=w338:T3)  [unwired: 9 in, 1 out]
      n132 = call <vilib>:"WPI_RelayRefNum Registry Get.vi"("refnum name"="Loader") -> ("RelayDevRef"=w340:T3)  [unwired: 9 in, 1 out]
      n133 = call <vilib>:"WPI_RelayRefNum Registry Get.vi"("refnum name"="SV 2") -> ("RelayDevRef"=w336:T3)  [unwired: 9 in, 1 out]
      n134 = flat-sequence {
        tunnel: [w373] -> w363
        tunnel: [w372] -> w362
        tunnel: [w371] -> w361
        tunnel: [w370] -> w360
        tunnel: [w368] -> w359
        tunnel: w342 -> [w367]
        tunnel: w340 -> [w366]
        tunnel: w338 -> [w365]
        tunnel: w336 -> [w364]
        tunnel: w363 -> [_]
        tunnel: w362 -> [w382]
        tunnel: w361 -> [w381]
        tunnel: w360 -> [w380]
        tunnel: w359 -> [w379]
        tunnel: [w382] -> w358
        tunnel: [w381] -> w357
        tunnel: [w380] -> w356
        tunnel: w358 -> [w411]
        tunnel: w357 -> [w410]
        tunnel: w356 -> [w409]
        tunnel: [w411] -> w355
        tunnel: [w410] -> w354
        tunnel: [w409] -> w353
        tunnel: w355 -> [w419]
        tunnel: w354 -> [w418]
        tunnel: w353 -> [w417]
        tunnel: [w416] -> w352
        tunnel: [w415] -> w351
        tunnel: [w414] -> w350
        tunnel: w352 -> [w429]
        tunnel: w351 -> [w428]
        tunnel: w350 -> [w427]
        tunnel: [w426] -> w349
        tunnel: [w425] -> w348
        tunnel: [w424] -> w347
        tunnel: w349 -> [w439]
        tunnel: w348 -> [w438]
        tunnel: w347 -> [w437]
        tunnel: [w436] -> w346
        tunnel: [w435] -> w345
        tunnel: [w434] -> w344
        tunnel: w346 -> [w449]
        tunnel: w345 -> [w448]
        tunnel: w344 -> [w447]
        tunnel: [w446] -> _
        tunnel: [w445] -> _
        tunnel: [w444] -> _
        frame #0 {
          # ".5 seconds"
          # "Charge 3 Cylinders and Loader Arm Down and Trigger In"
          n135 = Wait (ms)(milliseconds to wait=u32 500) -> ()  [unwired: 1 out]
          n136 = call <vilib>:"WPI_RelaySet.vi"("RelayValue"=WPI_RelayValue."On", "RelayDevRef"=w364) -> ("RelayDevRef"=w372:T3)  [unwired: 8 in, 1 out]
          n137 = call <vilib>:"WPI_RobotDriveRefNum Registry Get.vi"("refnum name"="Four Motors") -> ("RobotDriveDevRef"=w368:T7)  [unwired: 1 in, 9 out]
          n138 = call <vilib>:"WPI_RelaySet.vi"("RelayValue"=WPI_RelayValue."Reverse", "RelayDevRef"=w367) -> ("RelayDevRef"=w371:T3)  [unwired: 8 in, 1 out]
          n139 = call <vilib>:"WPI_RelaySet.vi"("RelayValue"=WPI_RelayValue."Reverse", "RelayDevRef"=w365) -> ("RelayDevRef"=w370:T3)  [unwired: 8 in, 1 out]
          n140 = call <vilib>:"WPI_RelaySet.vi"("RelayValue"=WPI_RelayValue."Forward", "RelayDevRef"=w366) -> ("RelayDevRef"=w373:T3)  [unwired: 8 in, 1 out]
        }
        frame #1 {
          # "Drive Forward"
          n141 = while {
            shift-right: [w394] -> _
            shift-left: w379 -> [w399]
            stop <- w387 stop-if-true
            w391 = 0.0 ("output")
            # "Drive To Target"
            n142 = Wait (ms)(milliseconds to wait=u32 50) -> ()  [unwired: 1 out]
            n143 = shared-variable ".\\Globals.lvlib\\Scores"() -> (w398:dbl)  [unwired: 1 in, 1 out]
            n144 = shared-variable ".\\Globals.lvlib\\Distance (ft)"() -> (w389:dbl)  [unwired: 1 in, 1 out]
            n145 = Less?(x=w398, y=50.0) -> (x < y?=w396:bool)
            n146 = case shown="False" w396 {
              tunnel: [w404 w407] -> w386
              tunnel: 10.5 ("setpoint") -> [w404 w407]
              tunnel: [w402 0.0 ("output")] -> w390
              tunnel: w389 -> [w400 w405]
              tunnel: [w400 w405] -> w388
              frame False {
                n147 = call-poly <vilib>:"PID.vi"("output range"=cluster{"output high":dbl, "output low":dbl} {"output high"=0.5, "output low"=-0.5}, "PID gains"=T1 {"proportional gain (Kc)"=0.28, "integral time (Ti, min)"=0.015, "derivative time (Td, min)"=1e-25} ("Distance Gains"), "process variable"=w400, "setpoint"=w404) -> ("output"=w402:dbl)  [unwired: 6 in, 1 out]
              }
              frame True {
              }
            }
            "Motor Outputs 2" <- w390
            n148 = Increment(x=w386) -> (x+1=w385:dbl)
            n149 = Decrement(x=w386) -> (x-1=w395:dbl)
            n150 = In Range and Coerce(upper limit=w385, x=w388, lower limit=w395) -> (In Range?=w387:bool)  [unwired: 1 out]
            n151 = Select(t=w391, s=w387, f=w390) -> (s? t:f=w384:dbl)
            n152 = Negate(x=w384) -> (-x=w383:dbl)
            n153 = call-poly <vilib>:"WPI_RobotDriveHolonomicDrive.vi"("Rotation"=w391, "Y"=w383, "X"=w391, "RobotDriveDevRef"=w399) -> ("RobotDriveDevRef"=w394:T7)  [unwired: 5 in, 2 out]
          }
        }
        frame #2 {
          n154 = shared-variable ".\\Globals.lvlib\\Hot or Not"() -> (w408:bool)  [unwired: 1 in, 1 out]
          n155 = case shown="True" w408 {
            frame False {
              n156 = Wait (ms)(milliseconds to wait=u32 1500) -> ()  [unwired: 1 out]
            }
            frame True {
              n157 = Wait (ms)(milliseconds to wait=u32 1) -> ()  [unwired: 1 out]
            }
          }
        }
        frame #3 {
          # "Release Trigger and Shoot"
          n158 = Wait (ms)(milliseconds to wait=u32 1500) -> ()  [unwired: 1 out]
          n159 = call <vilib>:"WPI_RelaySet.vi"("RelayValue"=WPI_RelayValue."Forward", "RelayDevRef"=w418) -> ("RelayDevRef"=w415:T3)  [unwired: 8 in, 1 out]
          n160 = call <vilib>:"WPI_RelaySet.vi"("RelayValue"=WPI_RelayValue."Reverse", "RelayDevRef"=w417) -> ("RelayDevRef"=w414:T3)  [unwired: 8 in, 1 out]
          n161 = call <vilib>:"WPI_RelaySet.vi"("RelayValue"=WPI_RelayValue."On", "RelayDevRef"=w419) -> ("RelayDevRef"=w416:T3)  [unwired: 8 in, 1 out]
        }
        frame #4 {
          # "Pull in Cylinders"
          n162 = Wait (ms)(milliseconds to wait=u32 3000) -> ()  [unwired: 1 out]
          n163 = call <vilib>:"WPI_RelaySet.vi"("RelayValue"=WPI_RelayValue."Off", "RelayDevRef"=w428) -> ("RelayDevRef"=w425:T3)  [unwired: 8 in, 1 out]
          n164 = call <vilib>:"WPI_RelaySet.vi"("RelayValue"=WPI_RelayValue."Off", "RelayDevRef"=w427) -> ("RelayDevRef"=w424:T3)  [unwired: 8 in, 1 out]
          n165 = call <vilib>:"WPI_RelaySet.vi"("RelayValue"=WPI_RelayValue."Off", "RelayDevRef"=w429) -> ("RelayDevRef"=w426:T3)  [unwired: 8 in, 1 out]
        }
        frame #5 {
          # "Lock Trigger"
          n166 = Wait (ms)(milliseconds to wait=u32 250) -> ()  [unwired: 1 out]
          n167 = call <vilib>:"WPI_RelaySet.vi"("RelayValue"=WPI_RelayValue."Reverse", "RelayDevRef"=w438) -> ("RelayDevRef"=w435:T3)  [unwired: 8 in, 1 out]
          n168 = call <vilib>:"WPI_RelaySet.vi"("RelayValue"=WPI_RelayValue."Off", "RelayDevRef"=w437) -> ("RelayDevRef"=w434:T3)  [unwired: 8 in, 1 out]
          n169 = call <vilib>:"WPI_RelaySet.vi"("RelayValue"=WPI_RelayValue."Off", "RelayDevRef"=w439) -> ("RelayDevRef"=w436:T3)  [unwired: 8 in, 1 out]
        }
        frame #6 {
          # "Turn off All"
          n170 = Wait (ms)(milliseconds to wait=u32 100) -> ()  [unwired: 1 out]
          n171 = call <vilib>:"WPI_RelaySet.vi"("RelayValue"=WPI_RelayValue."Off", "RelayDevRef"=w448) -> ("RelayDevRef"=w445:T3)  [unwired: 8 in, 1 out]
          n172 = call <vilib>:"WPI_RelaySet.vi"("RelayValue"=WPI_RelayValue."Off", "RelayDevRef"=w447) -> ("RelayDevRef"=w446:T3)  [unwired: 8 in, 1 out]
          n173 = call <vilib>:"WPI_RelaySet.vi"("RelayValue"=WPI_RelayValue."Off", "RelayDevRef"=w449) -> ("RelayDevRef"=w444:T3)  [unwired: 8 in, 1 out]
        }
      }
    }
  }
  n174 = call <vilib>:"WPI_JoystickGet.vi"("JoystickDevRef"=w7) -> ("Axes"=w5:T16)  [unwired: 1 in, 5 out]
  n175 = Unbundle By Name(w5) -> ()  [unwired: 1 out]
  n176 = Cluster To Array(cluster=w5) -> (array=w6:dbl[])
  n177 = call <vilib>:"SD Write Numeric Array.vi"("Numeric Array"=w6, "Name"="Joystick 1/Axes") -> ()  [unwired: 8 in, 2 out]
